vi "configuration UI.vi"() -> ()   [LabVIEW 2013, in "EthernetIP editor node.lvclass"]
uses:
  EthernetIP editor node.lvclass
  <vilib>/CEF_TreeControl/Node/NodeRef.ctl
  <vilib>/CEF_TreeControl/Node/NISE_CEF_Node.lvclass
  <vilib>/NI/AMC/Message Queue.ctl
  <vilib>/NI/AMC/Message.ctl
  <vilib>/NI/Tools/Keyed Array/KeyedArray.ctl
  <vilib>/CEF_TreeControl/Node/UserEventRef.ctl
  <vilib>/CEF_TreeControl/Controls/EventCluster.ctl
  <vilib>/NI/TBM Modules/Ethernet IP/configuration/EthernetIP configuration.lvclass
  <vilib>/NI/Module Execution Interface/Engine Configuration/engine configuration.lvclass
  <vilib>/NI/Tag Bus Data Framework/Configuration Editor/Classes/Engine Parent/Engine Parent Editor Node.lvclass
  <vilib>/NI/Tag Bus/tag/tag descriptor.lvclass
  <vilib>/NI/Tag Bus/tag/Data Type.ctl
  <vilib>/NI/Tag Bus/tag/tag descriptor.lvclass/tag descriptor.ctl
  <vilib>/NI/Tag Bus Module Framework/root configuration/TBM configuration.lvclass/TBM configuration.ctl
  <vilib>/NI/TBM Modules/Ethernet IP/configuration/EthernetIP configuration.lvclass/EthernetIP configuration.ctl
  <vilib>/NI/TBM Modules/Ethernet IP/configuration/assembly definition.ctl
  <vilib>/NI/TBM Modules/Ethernet IP/configuration/assembly type.ctl
  <vilib>/NI/Tag Bus/tag/write tag name.vi
  <vilib>/NI/Tag Bus/tag/write data type.vi
  <vilib>/NI/TBM Modules/Ethernet IP/configuration/Read assemblies.vi
  <vilib>/NI/Tag Bus Module Framework/root configuration/Read instance name.vi
  <vilib>/NI/Tag Bus Data Framework/Configuration Editor/Classes/Module editor node/Read Module Configuration.vi
  <vilib>/NI/Tag Bus Module Framework/root configuration/create GUID.vi
  <vilib>/NI/Tag Bus Module Framework/root configuration/TBM configuration.lvclass
  <vilib>/NI/Tag Bus Module Framework/module configuration/TBM module configuration.lvclass
  <vilib>/CEF_TreeControl/NISE_CEF_TreeControl.lvlib
  <vilib>/NI/Tag Bus Data Framework/Configuration Editor/Classes/Module editor node/module editor node.lvclass
  <vilib>/NI/TBM Modules/Ethernet IP/channel/EthernetIP Channel.lvclass
  <vilib>/NI/Tools/Keyed Array/Tools_KeyedArray.lvlib
  <vilib>/NI/AMC/AMC.lvlib
panel:
  in  "Tab Control":enum32{"Assemblies", "Channels"}(tab)
  in  "Configure Assembly":bool
  in  "Remove Assembly":bool
  in  "Add Assembly":bool
  in  "assemblies":i32(listbox)
  in  "Remove Button":bool
  in  "Add Button":bool
  in  "channel":i32(listbox)
  in  "settings":bool
  in  "user event":T1
  in  "main queue":T2
  in  "node ref":T3
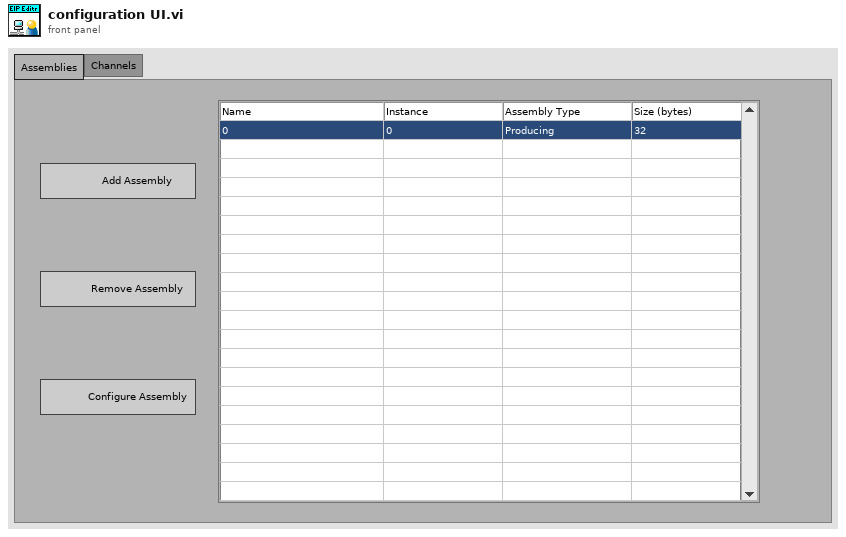
[diagram p1: front panel]
types:
  T1 = typedef "NISE_CEF_Node.lvclass/UserEventRef.ctl" = refnum<user-event>
  T2 = typedef "AMC.lvlib/Message Queue.ctl" = refnum<queue>
  T3 = typedef "NISE_CEF_Node.lvclass/NodeRef.ctl" = refnum<data-value>
  T4 = typedef "tag bus.lvlib/tag descriptor.lvclass/Data Type.ctl" = enum16{"Double", "Single", "I64", "I32", "I16", "I8", "U64", "U32", "U16", "U8", "Boolean", "String", "Array of Double", "Array of Single", "Array of I64", "Array of I32", "Array of I16", "Array of I8", "Array of U64", "Array of U32", "Array of U16", "Array of U8", "Array of Boolean", "Array of String"}
  T5 = typedef "NISE_CEF_TreeControl.lvlib/EventCluster.ctl" = cluster{"command":string, "data":string}
  T6 = typedef "EthernetIP configuration.lvclass/assembly definition.ctl" = cluster{"name":string, "Instance ID":u32, "Type":T7, "Size (bytes)":u32}
  T7 = typedef "EthernetIP configuration.lvclass/assembly type.ctl" = enum32{"Producing", "Consuming"}
  T8 = typedef "EthernetIP editor node.lvclass/table line.ctl" = cluster{"eip channels":refnum<class "EthernetIP Channel.lvclass">, "tag name":string}
  T9 = typedef "LVPoint32TypeDef.ctl" = cluster{"Horizontal":i32, "Vertical":i32}
  T10 = typedef "LVRowAndColumnTypeDef.ctl" = cluster{"Row":i32, "Column":i32}
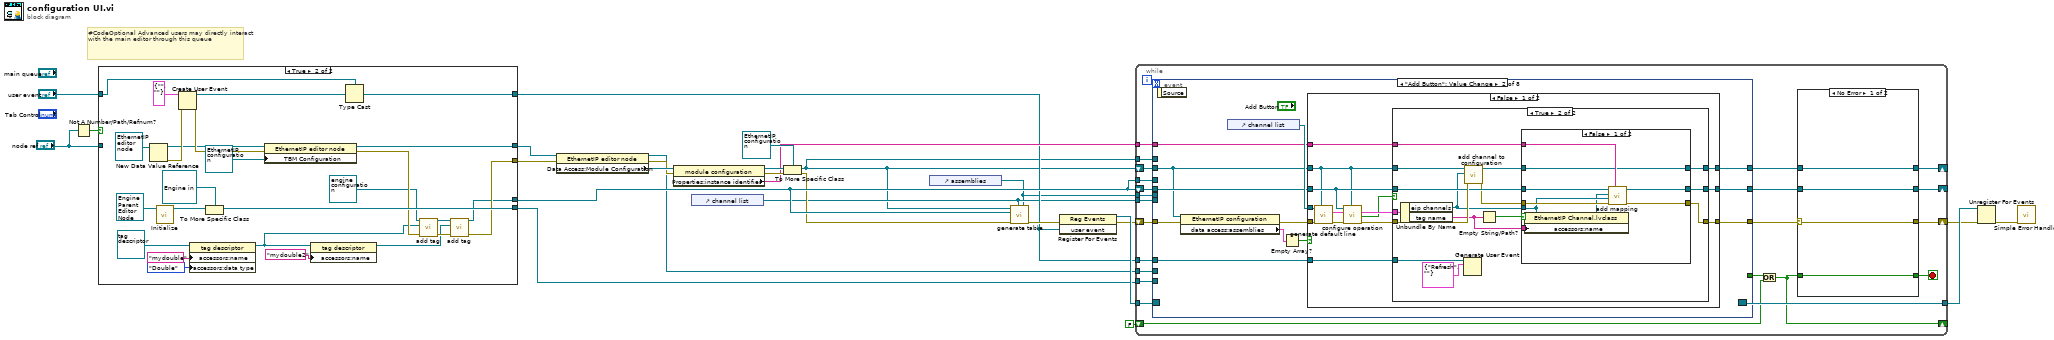
[diagram p0: block diagram]
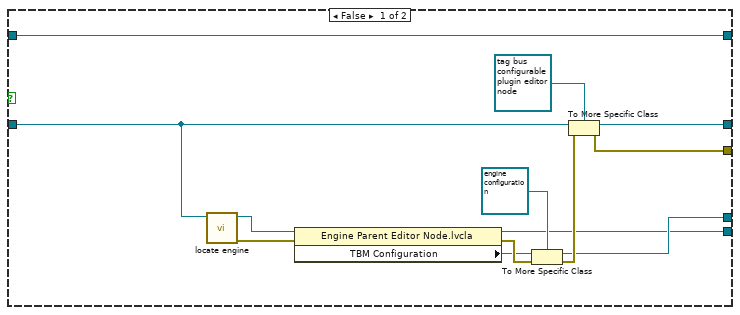
[diagram p2: hidden frame]
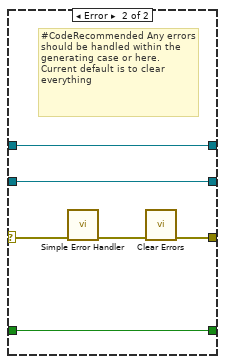
[diagram p3: hidden frame]
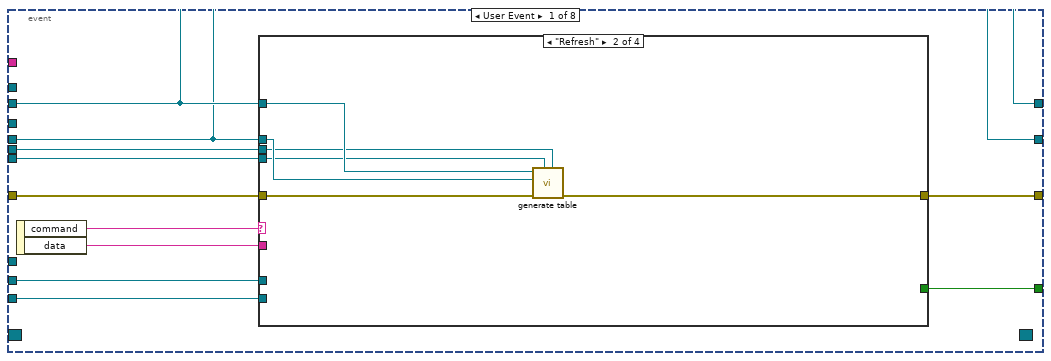
[diagram p4: hidden frame]
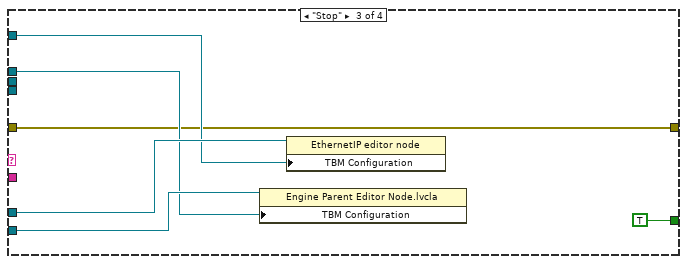
[diagram p6: hidden frame]
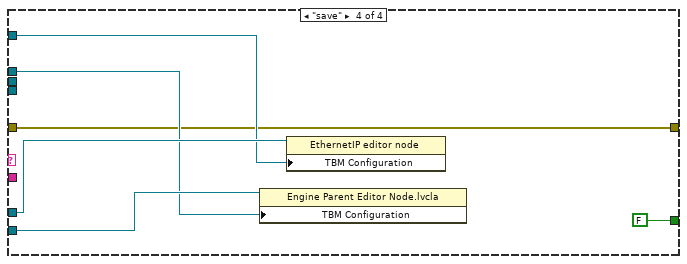
[diagram p7: hidden frame]
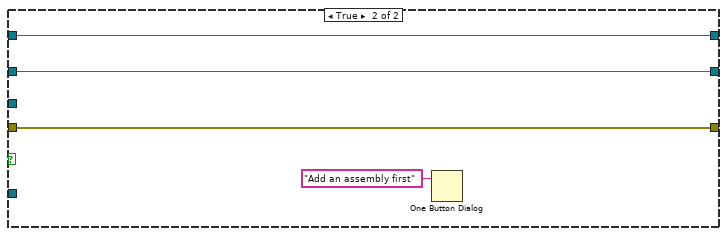
[diagram p10: hidden frame]
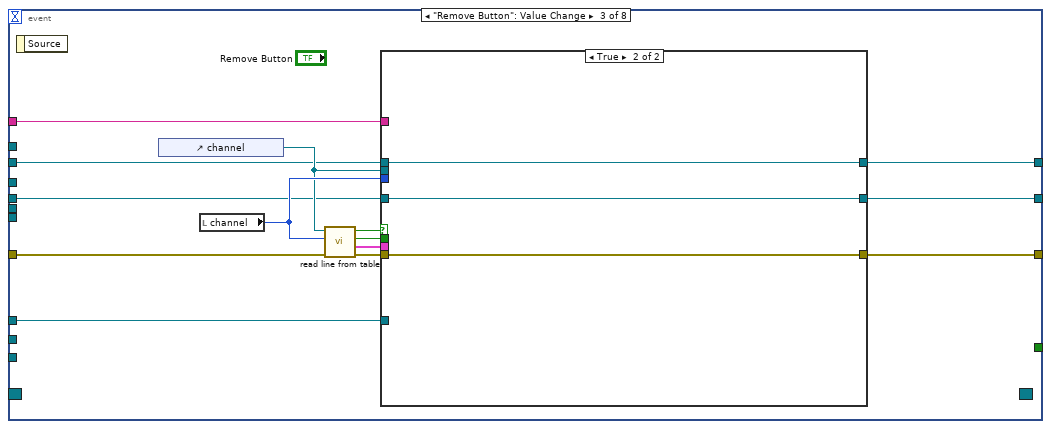
[diagram p11: hidden frame]
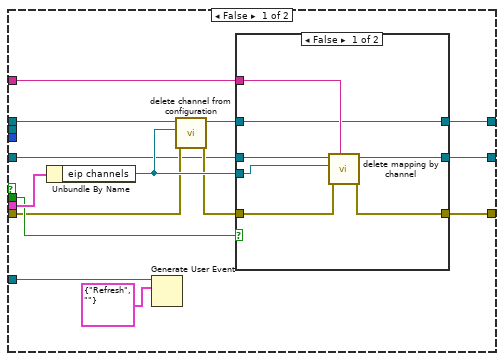
[diagram p12: hidden frame]
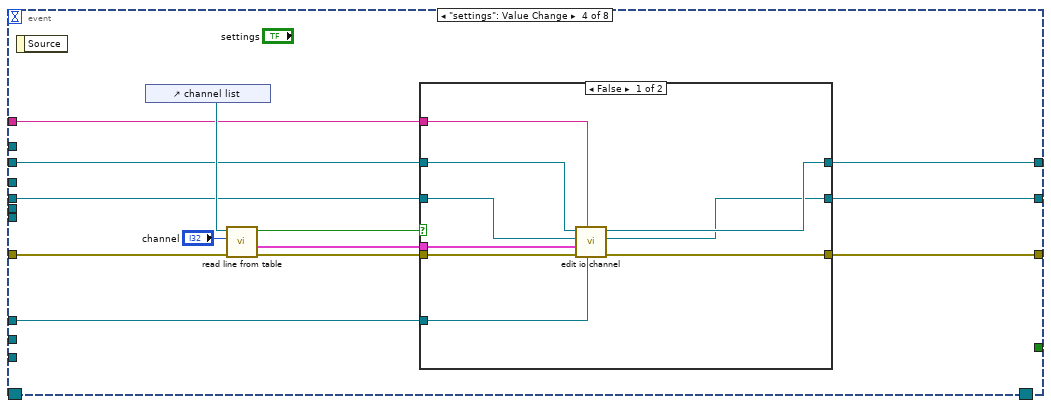
[diagram p14: hidden frame]
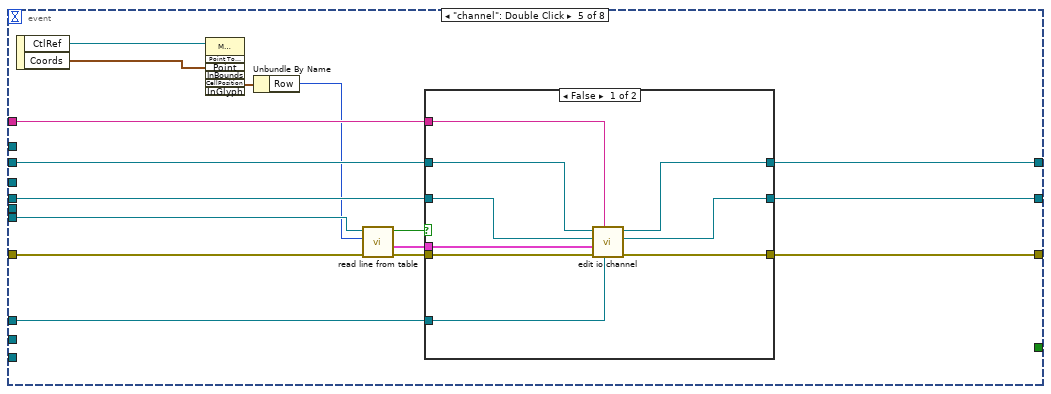
[diagram p16: hidden frame]
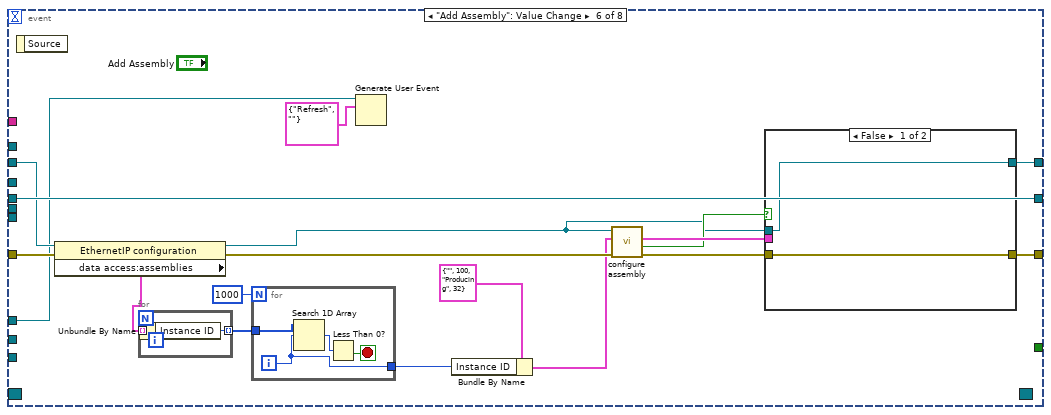
[diagram p18: hidden frame]
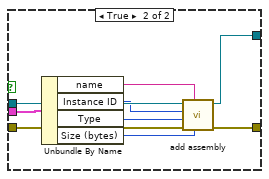
[diagram p19: hidden frame]
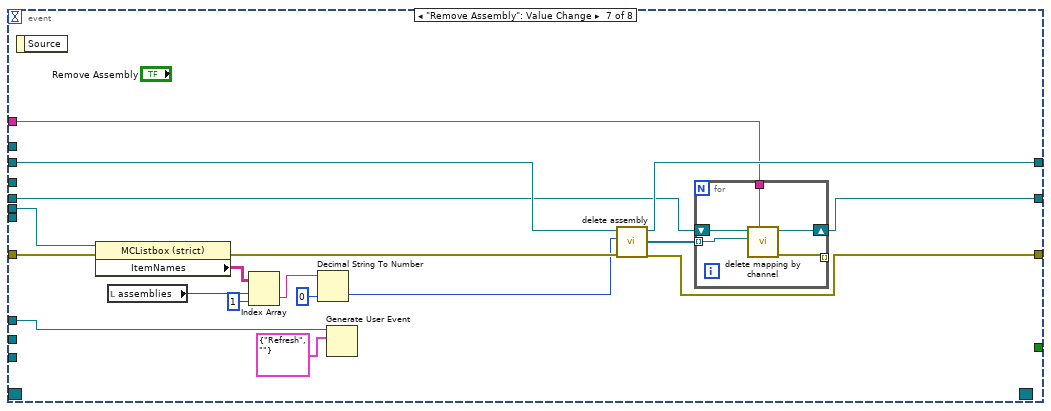
[diagram p20: hidden frame]
diagram:
  # "#CodeOptional Advanced users may directly interact with the main editor through this queue"
  n1 = Not A Number/Path/Refnum?(number/path/refnum="node ref") -> (NaN/Path/Refnum?=w17:bool)
  n2 = case shown="True" w17 {
    tunnel: "user event" -> [w39 w41]
    tunnel: [w39 w42] -> w4
    tunnel: "node ref" -> [w37 _]
    tunnel: [w36 w59] -> w10
    tunnel: [w35 w46] -> w15
    tunnel: [w28 w45] -> w12
    tunnel: [w27 w56] -> w6
    frame False {
      n3 = call <vilib>:"locate engine.vi"("component"=w37) -> ("error out"=w32:errorcluster, "engine"=w34:refnum<data-value>)  [unwired: 9 in]
      n4 = property class="Engine Parent Editor Node.lvcla"(reference=w34, error in=w32) -> (reference out=w27:refnum<data-value>, error out=w31:errorcluster, "TBM Configuration"=w30:refnum<class "TBM configuration.lvclass">)
      n5 = To More Specific Class(target class=refnum<class "engine configuration.lvclass"> refnum ("engine configuration.lvclass"), reference=w30, error in=w31) -> (specific class reference=w28:refnum<class "engine configuration.lvclass">, error out=w29:errorcluster)
      n6 = To More Specific Class(target class=refnum<data-value> refnum ("data value reference"), reference=w37, error in=w29) -> (specific class reference=w36:refnum<data-value>, error out=w35:errorcluster)
    }
    frame True {
      n7 = New Data Value Reference(data value=refnum<class "EthernetIP editor node.lvclass"> refnum ("tag bus configurable plugin editor node")) -> (data value reference=w58:refnum<data-value>, error out=w61:errorcluster)  [unwired: 1 in]
      n8 = call-dynamic "Initialize.vi"("Engine in"=refnum<class "Engine Parent Editor Node.lvclass"> refnum) -> ("data value reference"=w57:T3)  [unwired: 8 in, 2 out]
      n9 = Create User Event(user event datatype=T5 {"command"="", "data"=""} ("event data"), error in=w61) -> (user event=w64:refnum<user-event>, error out=w60:errorcluster)
      n10 = property class="tag descriptor"(reference=refnum<class "tag descriptor.lvclass"> refnum ("tag descriptor"), "accessors:name"="mydouble" ("name"), "accessors:data type"=Data_Type."Double" ("data type")) -> (reference out=w43:refnum<class "tag descriptor.lvclass">)  [unwired: 1 in, 1 out]
      n11 = To More Specific Class(target class=refnum<data-value> refnum ("data value reference"), reference=w57) -> (specific class reference=w56:refnum<data-value>)  [unwired: 1 in, 1 out]
      n12 = property class="EthernetIP editor node"(reference=w58, error in=w60, "TBM Configuration"=refnum<class "EthernetIP configuration.lvclass"> refnum ("tag bus configurable plugin module configuration")) -> (reference out=w59:refnum<data-value>, error out=w50:errorcluster)
      n13 = property class="tag descriptor"(reference=w43, "accessors:name"="mydouble2" ("name")) -> (reference out=w44:refnum<class "tag descriptor.lvclass">)  [unwired: 1 in, 1 out]
      n14 = Type Cast(type=w41, x=w64) -> (*(type *) &x=w42:T1)
      n15 = call <vilib>:"add tag.vi"("error in"=w50, "tag descriptor"=w43, "engine configuration in"=refnum<class "engine configuration.lvclass"> refnum ("Engine Configuration")) -> ("error out"=w48:errorcluster, "engine configuration out"=w47:refnum<class "engine configuration.lvclass">)  [unwired: 7 in]
      n16 = call <vilib>:"add tag.vi"("error in"=w48, "tag descriptor"=w44, "engine configuration in"=w47) -> ("error out"=w46:errorcluster, "engine configuration out"=w45:refnum<class "engine configuration.lvclass">)  [unwired: 7 in]
    }
  }
  n17 = property class="EthernetIP editor node"(reference=w10, error in=w15) -> (reference out=w7:refnum<data-value>, error out=w20:errorcluster, "Data Access:Module Configuration"=w21:refnum<class "TBM module configuration.lvclass">)
  n18 = property class="module configuration"(reference=w21, error in=w20) -> (reference out=w18:refnum<class "TBM module configuration.lvclass">, error out=w19:errorcluster, "Properties:instance identifier"=w14:string)
  n19 = control-ref of="channel list"() -> (w3:refnum<vi>)
  n20 = To More Specific Class(target class=refnum<class "EthernetIP configuration.lvclass"> refnum ("tag bus configurable plugin module configuration"), reference=w18, error in=w19) -> (specific class reference=w2:refnum<class "EthernetIP configuration.lvclass">, error out=w11:errorcluster)
  n21 = control-ref of="assemblies"() -> (w1:refnum<vi>)
  n22 = call "generate table.vi"("assemblies"=w1, "table"=w3, "error in"=w11, "engine configuration in"=w12, "EthernetIP configuration in"=w2) -> ("error out"=w9:errorcluster)  [unwired: 6 in]
  n23 = register-events(error in=w9, w4) -> (reference out=w26:refnum<event-registration>, error out=w8:errorcluster)  [unwired: 1 in]
  n24 = while {
    tunnel: w26 -> [w88]
    tunnel: [w87] -> w25
    shift-right: [w81] -> w24
    shift-left: w8 -> [w86]
    shift-right: [w83] -> _
    shift-left: FALSE -> [w82]
    tunnel: w2 -> [w79]
    shift-right: [w75] -> _
    shift-left: w2 -> [w80]
    shift-right: [w76] -> _
    shift-left: w12 -> [w77]
    tunnel: w12 -> [w78]
    tunnel: w14 -> [w74]
    tunnel: w7 -> [w71]
    tunnel: w6 -> [w70]
    tunnel: w4 -> [w69]
    tunnel: w3 -> [w67]
    tunnel: w1 -> [w66]
    stop <- w85 stop-if-true
    n25 = event shown="[1] \"Add Button\": Value Change" {
      selector: w88 -> [_ _ _ _ _ _ _ _]
      dyn-events: [_ _ _ _ _ _ _ _] -> w87
      timeout: _ -> [_ _ _ _ _ _ _ _]
      tunnel: [w109 _ _ _ _ _ _ _] -> w84
      tunnel: [w101 w140 w202 w241 w269 w297 w318 w350] -> w68
      tunnel: w86 -> [w102 w139 w201 w242 w270 w300 w335 w360]
      tunnel: w80 -> [w105 w130 w197 w235 w265 w292 w327 w349]
      tunnel: w79 -> [_ _ _ _ _ _ _ _]
      tunnel: w78 -> [_ _ _ _ _ _ _ _]
      tunnel: w77 -> [w104 w137 w196 w236 w266 w299 w323 w345]
      tunnel: [w104 w136 w191 w233 w263 w299 w322 w344] -> w73
      tunnel: [w105 w135 w190 w234 w264 w296 w326 w348] -> w72
      tunnel: w74 -> [_ w134 w192 w232 w262 _ w321 w343]
      tunnel: w71 -> [w107 _ _ _ _ _ _ _]
      tunnel: w70 -> [w106 _ _ _ _ _ _ _]
      tunnel: w69 -> [_ w133 w189 w231 w261 w284 w319 w341]
      tunnel: w67 -> [w100 _ _ _ w260 _ _ _]
      tunnel: w66 -> [w99 _ _ _ _ _ w333 w359]
      event User Event {
        n26 = event-data() -> ("command"=w108:string, "data"=w103:string)  [unwired: 1 in]
        n27 = case shown="\"Refresh\"" w108 {
          tunnel: [_ _ TRUE FALSE] -> w109
          tunnel: w107 -> [_ _ w121 w127]
          tunnel: w106 -> [_ _ w120 w126]
          tunnel: w105 -> [_ w116 w119 w125]
          tunnel: w104 -> [_ w115 w118 w124]
          tunnel: w103 -> [_ _ _ _]
          tunnel: w102 -> [w110 w114 w117 w123]
          tunnel: [w110 w113 w117 w123] -> w101
          tunnel: w100 -> [_ w112 _ _]
          tunnel: w99 -> [_ w111 _ _]
          frame Default {
          }
          frame "Refresh" {
            n28 = call "generate table.vi"("assemblies"=w111, "table"=w112, "error in"=w114, "engine configuration in"=w115, "EthernetIP configuration in"=w116) -> ("error out"=w113:errorcluster)  [unwired: 6 in]
          }
          frame "Stop" {
            n29 = property class="Engine Parent Editor Node.lvcla"(reference=w120, "TBM Configuration"=w118) -> ()  [unwired: 1 in, 2 out]
            n30 = property class="EthernetIP editor node"(reference=w121, "TBM Configuration"=w119) -> ()  [unwired: 1 in, 2 out]
          }
          frame "save" {
            n31 = property class="Engine Parent Editor Node.lvcla"(reference=w126, "TBM Configuration"=w124) -> ()  [unwired: 1 in, 2 out]
            n32 = property class="EthernetIP editor node"(reference=w127, "TBM Configuration"=w125) -> ()  [unwired: 1 in, 2 out]
          }
        }
      }
      event "Add Button": Value Change {
        n33 = event-data() -> ()  [unwired: 1 in, 1 out]
        n34 = property class="EthernetIP configuration"(reference=w130, error in=w139) -> (error out=w131:errorcluster, "data access:assemblies"=w129:T6[])  [unwired: 1 out]
        n35 = control-ref of="channel list"() -> (w138:refnum<vi>)
        n36 = Empty Array?(array=w129) -> (empty?=w132:bool)
        n37 = case shown="False" w132 {
          tunnel: [w154 w187] -> w140
          tunnel: w131 -> [w153 w187]
          tunnel: w138 -> [w152 _]
          tunnel: w130 -> [w141 w185]
          tunnel: w137 -> [w142 w186]
          tunnel: [w147 w186] -> w136
          tunnel: [w146 w185] -> w135
          tunnel: w134 -> [w145 _]
          tunnel: w133 -> [w143 _]
          frame False {
            n38 = call "generate default line.vi"("EthernetIP configuration"=w141, "error in"=w153, "operations table"=w152) -> ("error out"=w150:errorcluster, "line"=w151:T8)  [unwired: 7 in]
            n39 = call "configure operation.vi"("EthernetIP configuration"=w141, "error in"=w150, "line item in"=w151, "engine configuration in"=w142) -> ("error out"=w148:errorcluster, "success"=w144:bool, "line item out"=w149:T8)  [unwired: 4 in, 1 out]
            n40 = case shown="True" w144 {
              tunnel: [w157 w160] -> w154
              tunnel: w148 -> [w157 w170]
              tunnel: w142 -> [w156 w168]
              tunnel: w149 -> [_ w171]
              tunnel: w141 -> [w155 w172]
              tunnel: [w156 w167] -> w147
              tunnel: [w155 w161] -> w146
              tunnel: w145 -> [_ w164]
              tunnel: w143 -> [_ w159]
              frame False {
              }
              frame True {
                n41 = Unbundle By Name(w171) -> ("eip channels"=w165:refnum<class "EthernetIP Channel.lvclass">, "tag name"=w163:string)
                n42 = Generate User Event(user event=w159, event data cluster=T5 {"command"="Refresh", "data"=""} ("event data")) -> ()  [unwired: 2 in, 2 out]
                n43 = call <vilib>:"add channel to configuration.vi"("error in"=w170, "TBM channel in"=w165, "EthernetIP configuration in"=w172) -> ("error out"=w166:errorcluster, "EthernetIP configuration out"=w162:refnum<class "EthernetIP configuration.lvclass">)  [unwired: 7 in]
                n44 = Empty String/Path?(string/path=w163) -> (empty?=w169:bool)
                n45 = case shown="False" w169 {
                  tunnel: w168 -> [w181 w184]
                  tunnel: [w180 w184] -> w167
                  tunnel: w166 -> [w179 w183]
                  tunnel: w165 -> [w177 _]
                  tunnel: w164 -> [w178 _]
                  tunnel: w163 -> [w176 _]
                  tunnel: [w174 w183] -> w160
                  tunnel: w162 -> [w173 w182]
                  tunnel: [w173 w182] -> w161
                  frame False {
                    n46 = property class="EthernetIP Channel.lvclass"(reference=w177, "accessors:name"=w176) -> (reference out=w175:refnum<class "EthernetIP Channel.lvclass">)  [unwired: 1 in, 1 out]
                    n47 = call <vilib>:"add mapping.vi"("owner ID"=w178, "error in"=w179, "channel"=w177, "tag descriptor"=w175, "engine configuration"=w181) -> ("error out"=w174:errorcluster, "engine configuration out"=w180:refnum<class "engine configuration.lvclass">)  [unwired: 5 in]
                  }
                  frame True {
                  }
                }
              }
            }
          }
          frame True {
            n48 = One Button Dialog(message="Add an assembly first") -> ()  [unwired: 1 in, 1 out]
          }
        }
      }
      event "Remove Button": Value Change {
        n49 = event-data() -> ()  [unwired: 1 in, 1 out]
        n50 = control-ref of="channel"() -> (w199:refnum<vi>)
        n51 = local read "channel"() -> (w200:i32)
        n52 = call "read line from table.vi"("error in"=w201, "line number"=w200, "channels table"=w199) -> ("error out"=w193:errorcluster, "line"=w198:T8, "empty tag?"=w194:bool, "empty channel?"=w195:bool)  [unwired: 5 in]
        n53 = case shown="True" w195 {
          tunnel: [w205 w228] -> w202
          tunnel: w200 -> [_ _]
          tunnel: w199 -> [_ _]
          tunnel: w198 -> [w216 _]
          tunnel: w197 -> [w214 w227]
          tunnel: w196 -> [w209 w229]
          tunnel: w194 -> [w215 _]
          tunnel: w193 -> [w212 w228]
          tunnel: w192 -> [w208 _]
          tunnel: [w207 w229] -> w191
          tunnel: [w206 w227] -> w190
          tunnel: w189 -> [w203 _]
          frame False {
            n54 = Unbundle By Name(w216) -> ("eip channels"=w213:refnum<class "EthernetIP Channel.lvclass">)
            n55 = Generate User Event(user event=w203, event data cluster=T5 {"command"="Refresh", "data"=""} ("event data")) -> ()  [unwired: 2 in, 2 out]
            n56 = call <vilib>:"delete channel from configuration.vi"("error in"=w212, "TBM channel in"=w213, "EthernetIP configuration in"=w214) -> ("error out"=w210:errorcluster, "EthernetIP configuration out"=w211:refnum<class "EthernetIP configuration.lvclass">)  [unwired: 7 in]
            n57 = case shown="False" w215 {
              tunnel: w213 -> [w222 _]
              tunnel: w211 -> [w217 w224]
              tunnel: w210 -> [w220 w225]
              tunnel: w209 -> [w223 w226]
              tunnel: w208 -> [w221 _]
              tunnel: [w219 w226] -> w207
              tunnel: [w218 w225] -> w205
              tunnel: [w217 w224] -> w206
              frame False {
                n58 = call <vilib>:"delete mapping by channel.vi"("owner ID"=w221, "error in"=w220, "channel"=w222, "engine configuration in"=w223) -> ("error out"=w218:errorcluster, "engine configuration out"=w219:refnum<class "engine configuration.lvclass">)  [unwired: 6 in]
              }
              frame True {
              }
            }
          }
          frame True {
          }
        }
      }
      event "settings": Value Change {
        n59 = event-data() -> ()  [unwired: 1 in, 1 out]
        n60 = control-ref of="channel list"() -> (w240:refnum<vi>)
        n61 = call "read line from table.vi"("error in"=w242, "line number"="channel", "channels table"=w240) -> ("error out"=w239:errorcluster, "line"=w238:T8, "empty channel?"=w230:bool)  [unwired: 5 in, 1 out]
        n62 = case shown="False" w230 {
          tunnel: [w251 w252] -> w241
          tunnel: w239 -> [w250 w252]
          tunnel: w238 -> [w249 _]
          tunnel: w236 -> [w248 w253]
          tunnel: w235 -> [w247 w254]
          tunnel: [w246 w254] -> w234
          tunnel: [w245 w253] -> w233
          tunnel: w232 -> [w244 _]
          tunnel: w231 -> [w243 _]
          frame False {
            n63 = call "edit io channel.vi"("user event"=w243, "Properties:instance identifier"=w244, "error in"=w250, "line"=w249, "engine configuration in"=w248, "EthernetIP configuration in"=w247) -> ("error out"=w251:errorcluster, "engine configuration out"=w245:refnum<class "engine configuration.lvclass">, "EthernetIP configuration out"=w246:refnum<class "EthernetIP configuration.lvclass">)  [unwired: 3 in]
          }
          frame True {
          }
        }
      }
      event "channel": Double Click {
        n64 = event-data() -> ("CtlRef"=w259:refnum<vi>, "Coords"=w258:T9)  [unwired: 1 in]
        n65 = invoke class="MCListbox (strict)" method="Point To Row Column"(reference=w259, "Point"=w258) -> ("CellPosition"=w257:T10)  [unwired: 5 in, 6 out]
        n66 = Unbundle By Name(w257) -> ("Row"=w256:i32)
        n67 = call "read line from table.vi"("error in"=w270, "line number"=w256, "channels table"=w260) -> ("error out"=w268:errorcluster, "line"=w267:T8, "empty channel?"=w255:bool)  [unwired: 5 in, 1 out]
        n68 = case shown="False" w255 {
          tunnel: [w279 w280] -> w269
          tunnel: w268 -> [w278 w280]
          tunnel: w267 -> [w277 _]
          tunnel: w266 -> [w276 w281]
          tunnel: w265 -> [w275 w282]
          tunnel: [w274 w282] -> w264
          tunnel: [w273 w281] -> w263
          tunnel: w262 -> [w272 _]
          tunnel: w261 -> [w271 _]
          frame False {
            n69 = call "edit io channel.vi"("user event"=w271, "Properties:instance identifier"=w272, "error in"=w278, "line"=w277, "engine configuration in"=w276, "EthernetIP configuration in"=w275) -> ("error out"=w279:errorcluster, "engine configuration out"=w273:refnum<class "engine configuration.lvclass">, "EthernetIP configuration out"=w274:refnum<class "EthernetIP configuration.lvclass">)  [unwired: 3 in]
          }
          frame True {
          }
        }
      }
      event "Add Assembly": Value Change {
        n70 = event-data() -> ()  [unwired: 1 in, 1 out]
        n71 = property class="EthernetIP configuration"(reference=w292, error in=w300) -> (reference out=w291:refnum<class "EthernetIP configuration.lvclass">, error out=w293:errorcluster, "data access:assemblies"=w289:T6[])
        n72 = for {
          tunnel: w289 -> [w302] mode=indexing
          tunnel: [w301] -> w288 mode=indexing
          n73 = Unbundle By Name(w302) -> ("Instance ID"=w301:u32)
        }
        n74 = for {
          N: 1000 -> [_]
          tunnel: w288 -> [w306]
          tunnel: [w303] -> w283
          i -> [w303]
          stop <- w305 stop-if-true
          n75 = Search 1D Array(1D array=w306, element=w303) -> (index of element=w304:i32)  [unwired: 1 in]
          n76 = Less Than 0?(x=w304) -> (x < 0?=w305:bool)
        }
        n77 = Generate User Event(user event=w284, event data cluster=T5 {"command"="Refresh", "data"=""} ("event data")) -> ()  [unwired: 2 in, 2 out]
        n78 = Bundle By Name(cluster=T6 {"name"="", "Instance ID"=100, "Type"=enum."Producing", "Size (bytes)"=32} ("assembly definition in"), "Instance ID"=w283) -> (w286:T6)
        n79 = call "configure assembly.vi"("error in"=w293, "assembly definition in"=w286, "EthernetIP configuration"=w291) -> ("error out"=w298:errorcluster, "success"=w294:bool, "assembly definition out"=w295:T6)  [unwired: 5 in, 1 out]
        n80 = case shown="False" w294 {
          tunnel: w298 -> [w307 w317]
          tunnel: [w307 w316] -> w297
          tunnel: [w308 w315] -> w296
          tunnel: w291 -> [w308 w314]
          tunnel: w295 -> [_ w313]
          frame False {
          }
          frame True {
            n81 = Unbundle By Name(w313) -> ("name"=w309:string, "Instance ID"=w310:u32, "Type"=w311:T7, "Size (bytes)"=w312:u32)
            n82 = call <vilib>:"add assembly.vi"("size (bytes)"=w312, "name"=w309, "error in"=w317, "Type"=w311, "instance ID"=w310, "EthernetIP configuration in"=w314) -> ("error out"=w316:errorcluster, "EthernetIP configuration out"=w315:refnum<class "EthernetIP configuration.lvclass">)  [unwired: 4 in]
          }
        }
      }
      event "Remove Assembly": Value Change {
        n83 = event-data() -> ()  [unwired: 1 in, 1 out]
        n84 = property class="MCListbox (strict)"(reference=w333, error in=w335) -> (error out=w334:errorcluster, "ItemNames"=w332:string[][])  [unwired: 1 out]
        n85 = local read "assemblies"() -> (w331:i32)
        n86 = Index Array(array=w332, index (row)=w331, index (col)=1 ("disabled index (col)")) -> (element=w329:string)
        n87 = Decimal String To Number(string=w329, default (0L)=u32 0 ("default (0 I32)")) -> (number=w325:u32)  [unwired: 1 in, 1 out]
        n88 = Generate User Event(user event=w319, event data cluster=T5 {"command"="Refresh", "data"=""} ("event data")) -> ()  [unwired: 2 in, 2 out]
        n89 = call <vilib>:"delete assembly.vi"("error in"=w334, "instance ID"=w325, "EthernetIP configuration in"=w327) -> ("error out"=w318:errorcluster, "invalidated channelsu"=w324:refnum<class "EthernetIP Channel.lvclass">[], "EthernetIP configuration out"=w326:refnum<class "EthernetIP configuration.lvclass">)  [unwired: 6 in]
        n90 = for {
          shift-right: [w340] -> w322
          shift-left: w323 -> [w339]
          tunnel: w321 -> [w338]
          tunnel: w324 -> [w337] mode=indexing
          tunnel: [w336] -> _ mode=indexing
          n91 = call <vilib>:"delete mapping by channel.vi"("owner ID"=w338, "channel"=w337, "engine configuration in"=w339) -> ("error out"=w336:errorcluster, "engine configuration out"=w340:refnum<class "engine configuration.lvclass">)  [unwired: 7 in]
        }
      }
      event "Configure Assembly": Value Change {
        n92 = event-data() -> ()  [unwired: 1 in, 1 out]
        n93 = property class="MCListbox (strict)"(reference=w359, error in=w360) -> (error out=w355:errorcluster, "ItemNames"=w358:string[][])  [unwired: 1 out]
        n94 = Index Array(array=w358, index (row)="assemblies") -> (element=w356:string[])  [unwired: 1 in]
        n95 = Generate User Event(user event=w341, event data cluster=T5 {"command"="Refresh", "data"=""} ("event data")) -> ()  [unwired: 2 in, 2 out]
        n96 = call "table line to assembly.vi"("ItemNames"=w356) -> ("assembly definition"=w347:T6)  [unwired: 10 in]
        n97 = call "configure assembly.vi"("error in"=w355, "assembly definition in"=w347, "EthernetIP configuration"=w349) -> ("error out"=w351:errorcluster, "success"=w354:bool, "assembly definition out"=w346:T6, "changed"=w353:bool)  [unwired: 5 in]
        n98 = And(x=w353, y=w354) -> (x .and. y?=w352:bool)
        n99 = case shown="True" w352 {
          tunnel: w351 -> [w363 w375]
          tunnel: [w363 w366] -> w350
          tunnel: w349 -> [w362 w374]
          tunnel: [w362 w373] -> w348
          tunnel: w347 -> [_ w372]
          tunnel: w346 -> [_ w371]
          tunnel: w345 -> [w361 w370]
          tunnel: [w361 w369] -> w344
          tunnel: w343 -> [_ w368]
          frame False {
          }
          frame True {
            n100 = call <vilib>:"modify assembly.vi"("error in"=w375, "new"=w371, "original"=w372, "EthernetIP configuration in"=w374) -> ("error out"=w366:errorcluster, "channel classification changed"=w364:refnum<class "EthernetIP Channel.lvclass">[], "invalidated channels"=w367:refnum<class "EthernetIP Channel.lvclass">[], "EthernetIP configuration out"=w373:refnum<class "EthernetIP configuration.lvclass">)  [unwired: 4 in]
            n101 = Build Array (concatenate)(w367, w364) -> (w365:refnum<class "EthernetIP Channel.lvclass">[])
            n102 = for {
              shift-right: [w380] -> w369
              shift-left: w370 -> [w379]
              tunnel: w368 -> [w378]
              tunnel: w365 -> [w377] mode=indexing
              tunnel: [w376] -> _ mode=indexing
              n103 = call <vilib>:"delete mapping by channel.vi"("owner ID"=w378, "channel"=w377, "engine configuration in"=w379) -> ("error out"=w376:errorcluster, "engine configuration out"=w380:refnum<class "engine configuration.lvclass">)  [unwired: 7 in]
            }
          }
        }
      }
    }
    n104 = Or(x=w84, y=w82) -> (x .or. y?=w83:bool)
    n105 = case shown="No Error" w68 {
      selector: w68 -> [w89 w97]
      tunnel: [w92 w98] -> w85
      tunnel: w83 -> [w92 w98]
      tunnel: [w89 w95] -> w81
      tunnel: w73 -> [w90 w94]
      tunnel: [w90 w94] -> w76
      tunnel: w72 -> [w91 w93]
      tunnel: [w91 w93] -> w75
      frame No Error {
      }
      frame Error {
        # "#CodeRecommended Any errors should be handled within the generating case or here. Current default is to clear everything"
        n106 = call <vilib>:"Simple Error Handler.vi"("error in (no error)"=w97) -> ("error out"=w96:errorcluster)  [unwired: 4 in, 4 out]
        n107 = call <vilib>:"Clear Errors.vi"("error in (no error)"=w96) -> ("error out"=w95:errorcluster)  [unwired: 6 in]
      }
    }
  }
  n108 = Unregister For Events(event registration refnum=w25, error in=w24) -> (error out=w5:errorcluster)
  n109 = call <vilib>:"Simple Error Handler.vi"("error in (no error)"=w5) -> ()  [unwired: 4 in, 5 out]
